vi "deadband.vi"(10 "Threshold":sgl, 11 "Input":sgl) -> (3 "Output":sgl)   [LabVIEW 2013]
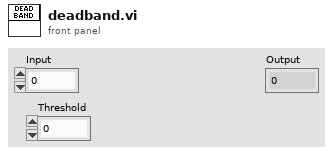
[diagram p1: front panel]
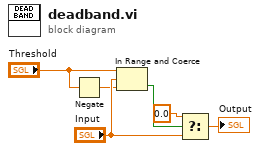
[diagram p0: block diagram]
diagram:
  n1 = Negate(x="Threshold") -> (-x=w2:sgl)
  n2 = In Range and Coerce(upper limit="Threshold", x="Input", lower limit=w2) -> (In Range?=w6:bool)  [unwired: 1 out]
  n3 = Select(t=sgl 0.0, s=w6, f="Input") -> (s? t:f=→"Output":sgl)
